vi "Trip Log and Trip Monitor.vi"(8 "error in (no error)":errorcluster, 11 "main ref":T1) -> (0 "error out":errorcluster)   [LabVIEW 2025]
uses:
  controls/LAB-IQ UI Data.ctl
  Traction Loop/Traction Receipe Enum.ctl
  <vilib>/Utility/error.llb/Trim Whitespace One-Sided.vi
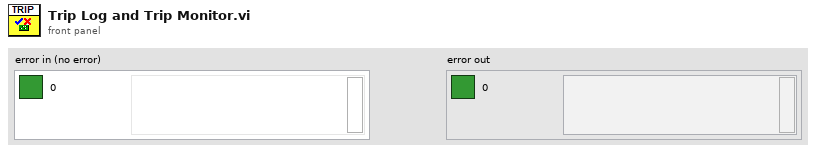
[diagram p1: front panel]
types:
  T1 = typedef "LAB-IQ UI Data.ctl" = cluster{"Main Home Screen":cluster{"GUI":refnum<vi>, "Platform Settings":refnum<vi>, "Configure":refnum<vi>, "Home":refnum<vi>, "EXIT":refnum<vi>, "service 2":refnum<vi>, "MainPage":refnum<vi>, "Analysis":refnum<vi>}, "Platform Settings":cluster{"mm/s  Surge":refnum<vi>, "Update Surge Speed":refnum<vi>, "Drive Error":refnum<vi>, "Disable Axis Jog Soft Limits":refnum<vi>, "mm/s  Sway":refnum<vi>, "Sway and Surge COM Status":refnum<vi>, "Heave COM Status":refnum<vi>, "Enable Platform":refnum<vi>, "Surge Forward Main":refnum<vi>, "Sway Right Main":refnum<vi>, "Sway Left Main":refnum<vi>, "Heave Down Main":refnum<vi>, "Heave Up main":refnum<vi>, "Update Sway Speed":refnum<vi>, "Update Heave Speed":refnum<vi>, "mm/s Heave":refnum<vi>, "mm/sec":refnum<vi>, "mm":refnum<vi>, "Surge Backward Main":refnum<vi>}, "Analysis Screen":cluster{"Analysis Home":refnum<vi>, "Surface Analysis":refnum<vi>, "Imaging":refnum<vi>, "Image Analysis":refnum<vi>, "Post Analysis":refnum<vi>}, "Config Screen":cluster{"Select Load Head":refnum<vi>, "Notes :":refnum<vi>, "FILE":refnum<vi>, "Sample ID :":refnum<vi>, "Operator ID :":refnum<vi>, "Operator Name :":refnum<vi>, "Auto":refnum<vi>}, "Motion Module":cluster{"zNL":refnum<vi>, "NL disp":refnum<vi>, "Rotary Tab":refnum<vi>, "Motion Direction:  3":refnum<vi>, "E.Velocity 2":refnum<vi>, "e.v/ssr 2":refnum<vi>, "Enter Fixed E.Velocity 2":refnum<vi>, "Enter Final SRR 2":refnum<vi>, "Enter initial SRR 2":refnum<vi>, "Enter Fixed SRR 2":refnum<vi>, "Enter the Final E.Velocity (m/s) 2":refnum<vi>, "Enter initial E.Velocity (m/s) 2":refnum<vi>, "Final Speed (RPM) 3":refnum<vi>, "Initial Speed (RPM) 2":refnum<vi>, "Enter the Final Velocity (m/s) 3":refnum<vi>, "Enter initial Velocity (m/s)  3":refnum<vi>, "Ramp Up 2":refnum<vi>, "TEST SELECTION":refnum<vi>, "SPEED SELECTION : ":refnum<vi>, "Angular Oscillation Set":refnum<vi>, "Traction":refnum<vi>, "Step Speed":refnum<vi>, "StepTable For Load-Speed":refnum<vi>, "StepTable For Speed":refnum<vi>, "Surge Forward MM":refnum<vi>, "Surge Backward MM":refnum<vi>, "M3 Image":refnum<vi>, "String 39":refnum<vi>, "Sway Left MM":refnum<vi>, "Sway Right MM":refnum<vi>, "Disable Axis Jog Soft Limits":refnum<vi>, "mm":refnum<vi>, "Heave Down MM":refnum<vi>, "Heave Up MM":refnum<vi>, "Wear Track Diameter (mm)":refnum<vi>, "Set WTD":refnum<vi>, "HomeScratch":refnum<vi>, "HomeRot":refnum<vi>, "PlaceModule":refnum<vi>, "Enter the Angle (Deg)":refnum<vi>, "Enter the Frequency (Hz)":refnum<vi>, "Motion Mode:":refnum<vi>, "LR Sway":refnum<vi>, "Rot Hor":refnum<vi>, "Scratch":refnum<vi>, "LR Cam":refnum<vi>, "MMBack":refnum<vi>, "MMNext":refnum<vi>, "Rot Ver":refnum<vi>, "Rotary Module Selection":refnum<vi>, "calculate rotary":refnum<vi>, "SPEED SELECTION : rotary":refnum<vi>, "Import 2":refnum<vi>, "Save 2":refnum<vi>, "File Path :  2":refnum<vi>, "String 45":refnum<vi>, "StepTable For Speed 3":refnum<vi>, "Enter the Speed(mm/sec)":refnum<vi>, "Enter the Speed(RPM)":refnum<vi>, "Enter Scratch Speed (mm/s):":refnum<vi>, "SwaySpeed Set":refnum<vi>, "Scartch Offset":refnum<vi>, "Motion type:":refnum<vi>, "HomeScratch 2":refnum<vi>, "Enter Scratch length (mm):":refnum<vi>, "Wear Track Diameter":refnum<vi>, "Rotary Speed Exced":refnum<vi>, "Scratch Mode":refnum<vi>, "No of Scratch":refnum<vi>}, "Environmental control":cluster{"Humidity  Status  3":refnum<vi>, "Low Temp  Status  2":refnum<vi>, "TK4 status 2":refnum<vi>, "Stage Temperature":refnum<vi>, "Sample Temperature":refnum<vi>, "Humidity (Amb)":refnum<vi>, "Clear List":refnum<vi>, "Add to list":refnum<vi>, "Wear":refnum<vi>, "Vibration":refnum<vi>, "Humidity (Chamber)":refnum<vi>, "Temperature (Chamber)":refnum<vi>, "ECR ":refnum<vi>, "Temperature (Amb)":refnum<vi>, "Microphone":refnum<vi>, "Acoustic Emission 3":refnum<vi>, "SNext":refnum<vi>, "APBack":refnum<vi>, "Enter the Temperature (°C):":refnum<vi>, "Enter the Stage \nTemperature (°C):":refnum<vi>, "Enter the Humidity (%Rh):":refnum<vi>, "Low Temp":refnum<vi>, "High Temp":refnum<vi>, "Humidity":refnum<vi>, "Sensors Picked":refnum<vi>}, "About Screen":cluster{"Password":refnum<vi>, "Home Service":refnum<vi>, "Advanced Setting":refnum<vi>, "About Tab":refnum<vi>, "ECR Port:":refnum<vi>, "Ramp Port:":refnum<vi>, "Installation/Replacement completed":refnum<vi>, "Loahead":refnum<vi>, "Heave and Surge COM Port:":refnum<vi>, "Sway COM Port:":refnum<vi>, "Temp Modbus:":refnum<vi>, "Humidity Port:":refnum<vi>, "Edit Gain Constants":refnum<vi>, "Save Gain Constants":refnum<vi>}, "Main Screen":cluster{"Main Screen Tab":refnum<vi>, "Angle and Frequency":refnum<vi>, "Stroke (mm)":refnum<vi>, "Angle (Deg)":refnum<vi>, "Main Speed Tab":refnum<vi>, "MTM MOTOR DISPLAY":refnum<vi>, "Disc Speed (m/sec)":refnum<vi>, "Ball Speed (m/sec)":refnum<vi>, "Disc Speed (RPM)":refnum<vi>, "Ball Speed (RPM)":refnum<vi>, "SPEED TAB":refnum<vi>, "Speed (m/sec)":refnum<vi>, "Set Speed (m/sec)":refnum<vi>, "Speed (RPM)":refnum<vi>, "Set Speed":refnum<vi>, "Time Tab":refnum<vi>, "Time ( HH:MM:SS ) 2":refnum<vi>, "Test Duration":refnum<vi>, "Test Duration 4":refnum<vi>, "TEST CYCLE":refnum<vi>, "TOTAL CYCLES":refnum<vi>, "Set Load (N)":refnum<vi>, "Temp Tabs":refnum<vi>, "Heater":refnum<vi>, "TK4 status":refnum<vi>, "ChamberTemp":refnum<vi>, "SetTmp":refnum<vi>, "Controller  Status":refnum<vi>, "ChamberTemp 2":refnum<vi>, "SetTmp 2":refnum<vi>, "Controller  Status 2":refnum<vi>, "ChamberTemp 3":refnum<vi>, "SetTmp 3":refnum<vi>, "Cooling":refnum<vi>, "Load Communication":refnum<vi>, "Ambient \nTemperature":refnum<vi>, "HumCOMStatus":refnum<vi>, "Ambient\n Humidity":refnum<vi>, "Freq (Hz)":refnum<vi>, "Load En":refnum<vi>, "NLt":refnum<vi>, "zNL 2":refnum<vi>, "Humidity On":refnum<vi>, "humidity disp":refnum<vi>, "Set Humidity":refnum<vi>, "NL disp 2":refnum<vi>, "Humidity On 2":refnum<vi>, "humidity disp 2":refnum<vi>, "Set Humidity 2":refnum<vi>, "NL disp 3":refnum<vi>, "AppLoadSeq scratch":refnum<vi>, "Stop Scratch":refnum<vi>, "ClrLog":refnum<vi>, "Trip Log":refnum<vi>, "STOP":refnum<vi>, "Start Test":refnum<vi>, "Test status":refnum<vi>, "AR Led":refnum<vi>, "Data":refnum<vi>, "Health":refnum<vi>, "Sway COM Status":refnum<vi>, "Heave COM Status":refnum<vi>, "Grp Tab":refnum<vi>, "Sub Graph":refnum<vi>, "SD (mm)":refnum<vi>, "Siliding distance Reset Graph":refnum<vi>, "SDGp":refnum<vi>, "Humidity Reset Graph":refnum<vi>, "HumrGp":refnum<vi>, "Acoustic Emission (mV)":refnum<vi>, "Aqucostic Reset Graph":refnum<vi>, "gACQUOS":refnum<vi>, "ECR RESET":refnum<vi>, "ECR":refnum<vi>, "Temperature Reset":refnum<vi>, "Acoustic Emission (mV) 2":refnum<vi>, "Aqucostic Reset Graph 2":refnum<vi>, "gACQUOS 2":refnum<vi>, "ECR RESET 2":refnum<vi>, "ECR 2":refnum<vi>, "Temperature Reset 2":refnum<vi>, "Temperature (deg c)":refnum<vi>, "Speed Reset Graph":refnum<vi>, "Speed Tab":refnum<vi>, "MTM DISC  SPEED":refnum<vi>, "MTM BALL SPEED":refnum<vi>, "speed mm/sec":refnum<vi>, "Hymidity":refnum<vi>, "Humidity Disable trip":refnum<vi>, "CoF Trip  2":refnum<vi>, "Depth Trip":refnum<vi>, "Weart Deapth":refnum<vi>, "Depth Reset Graph":refnum<vi>, "Weart":refnum<vi>, "Depthz":refnum<vi>, "Depth (µm)":refnum<vi>, "WearGp":refnum<vi>, "NL Trip 2":refnum<vi>, "Load pid":refnum<vi>, "Load Disable Trip":refnum<vi>, "Load Reset Graph":refnum<vi>, "NL Display 4":refnum<vi>, "Main Chart 3":refnum<vi>, "BACK":refnum<vi>, "Depth Trip 2":refnum<vi>, "COF TRIP ":refnum<vi>, "Friction Force (N)":refnum<vi>, "FF Reset Graph":refnum<vi>, "FF Disable Trip":refnum<vi>, "FF TRIP":refnum<vi>, "COF Disable Trip":refnum<vi>, "COF Reset Graph":refnum<vi>, "Start Test Temp":refnum<vi>, "zFF":refnum<vi>, "Friction Force (N) Graph":refnum<vi>, "Coefficient of Friction":refnum<vi>, "Scratch Start Test":refnum<vi>, "FF Tab":refnum<vi>, "Cyclic Friction Force (N)":refnum<vi>, "CZ FF":refnum<vi>, "Cyclic Friction Force (N) Graph":refnum<vi>, "Cyclic Coefficient of Friction":refnum<vi>, "Cyclic FF TRIP":refnum<vi>, "Cyclic FF Disable Trip":refnum<vi>, "cyclic COF Disable Trip":refnum<vi>, "cyclic COF TRIP":refnum<vi>, "cyclic COF Reset Graph":refnum<vi>, "Cyclic FF Reset Graph":refnum<vi>, "Test Trip":refnum<vi>, "Multi Scratch Pass":refnum<vi>, "Scratch Start Recording":refnum<vi>}, "Loading":cluster{"Indentation":refnum<vi>, "Reference Sample":refnum<vi>, "Load Cell Communication Slide":refnum<vi>, "com 3":refnum<vi>, "com":refnum<vi>, "DecaForce COM Status":refnum<vi>, "Update":refnum<vi>, "Clear 3":refnum<vi>, "seq":refnum<vi>, "Stribeck table":refnum<vi>, "Stribeck Table  For loading":refnum<vi>, "Loading Mode":refnum<vi>, "Enter the Final Load (N)":refnum<vi>, "Enter the CoF Trip":refnum<vi>, "Enter the Friction Force Trip":refnum<vi>, "Enter the Normal load Trip":refnum<vi>, "Enter the Load  (N)":refnum<vi>, "KiloForce":refnum<vi>, "DecaForce ":refnum<vi>, "MicroForce":refnum<vi>, "LHBack":refnum<vi>, "LHNext":refnum<vi>, "Enter the Loading Rate (N/min)":refnum<vi>, "Message":refnum<vi>, "Warning 2":refnum<vi>, "SSP 0.75":refnum<vi>, "SSP 0.5":refnum<vi>, "SSP 0.3":refnum<vi>, "Warning":refnum<vi>, "gui GIF":refnum<vi>, "Communication is established":refnum<vi>, "AppLoad 4":refnum<vi>, "Multipoint":refnum<vi>, "Load Selection":refnum<vi>}, "PID":cluster{"Ramp MulFac":refnum<vi>, "pulses LoadDiffRamp(2..10)":refnum<vi>, "PulseControlRamp(diff<=3N)":refnum<vi>, "SetLoadDeadband(%) Load(0-10N)":refnum<vi>, "PID gains out delay (microForce)":refnum<vi>, "Ramp":refnum<vi>, "Gain 2":refnum<vi>, "pulses LoadDiff(2..10)":refnum<vi>, "pulses LoadDiff(11..50)":refnum<vi>, "PulseControl(diff<=3N)":refnum<vi>, "SetLoadDeadband(%)  2":refnum<vi>, "Dummy Run":refnum<vi>, "Vertical load (N)":refnum<vi>, "AutoTune":refnum<vi>, "Offset 3 ":refnum<vi>, "apply load":refnum<vi>, "Offset  3":refnum<vi>, "apply load 2":refnum<vi>, "Enter ByPass Load":refnum<vi>, "reinit 3":refnum<vi>, "output range delay":refnum<vi>, "PID gains out delay":refnum<vi>, "Bypass Load":refnum<vi>, "pulsesSent":refnum<vi>, "pulses ":refnum<vi>, "actpid":refnum<vi>, "gFF Rot":refnum<vi>, "pulses LoadDiff(21..1000)":refnum<vi>, "Delay":refnum<vi>, "deadband":refnum<vi>}, "Config Parameters":cluster{"Tab Control 3":refnum<vi>, "Tab Control 19":refnum<vi>, "SAMPLES":refnum<vi>, "Re-initilaize":refnum<vi>, "Filter ON/OFF":refnum<vi>, "TracHomeSurgeOffsetCounts 10MM":refnum<vi>, "TracHomeSwayOffsetCounts 10MM":refnum<vi>, "Acoustic Emission:":refnum<vi>, "Apply Filter (FF)":refnum<vi>, "Filter% 2":refnum<vi>, "Apply Filter (Load)":refnum<vi>, "Filter% ":refnum<vi>, "Sway distance (mm)":refnum<vi>, "Surge distance (mm)":refnum<vi>, "DataSavingLoopDelay(ms)":refnum<vi>, "SAVE 2":refnum<vi>, "Enter Distance":refnum<vi>, "Sway Counts:":refnum<vi>, "Distance (mm): 3":refnum<vi>, "Surge Counts:":refnum<vi>, "Distance (mm): 2":refnum<vi>, "Distance (mm):":refnum<vi>, "Heave Counts:":refnum<vi>, "LRMHomeSurgeOffsetCounts":refnum<vi>, "LRMHomeSwayOffsetCounts":refnum<vi>, "TracHomeSurgeOffsetCounts 20MM":refnum<vi>, "TracHomeSwayOffsetCounts 20MM":refnum<vi>, "RotHomeSwayOffsetCounts":refnum<vi>, "RotHomeSurgeOffsetCounts":refnum<vi>, "Heave distance":refnum<vi>, "Zmm":refnum<vi>, "Heave Pulses/mm":refnum<vi>, "Surge Pulses/mm":refnum<vi>, "Sway Pulses/mm":refnum<vi>, "Heave Pitch":refnum<vi>, "Surge Pitch":refnum<vi>, "Sway Pitch":refnum<vi>, "Heave PPR":refnum<vi>, "Surge PPR":refnum<vi>, "Sway PPR":refnum<vi>, "Tab Control 5":refnum<vi>, "Tab Control 14":refnum<vi>, "Tab Control 26":refnum<vi>, "AE":refnum<vi>, "Heave Loop Delay":refnum<vi>, "Heave PID Speed":refnum<vi>, "Surge Jog Speed":refnum<vi>, "Heave Jog Speed":refnum<vi>, "Sway Loop Delay":refnum<vi>, "Sway PID Speed":refnum<vi>, "Sway Jog Speed":refnum<vi>, "DEPTH TRIP VALUE":refnum<vi>, "LOAD TRIP VALUE":refnum<vi>, "DEPTH TRIP   ENABLE":refnum<vi>, "LOAD TRIP  ENABLE":refnum<vi>, "CYCLIC FF TRIP VALUE":refnum<vi>, "FF TRIP VALUE":refnum<vi>, "CYCLIC CoF TRIP VALUE":refnum<vi>, "COF TRIP VALUE":refnum<vi>, "CYCLIC COF TRIP  ENABLE":refnum<vi>, "CYCLIC FF TRIP  ENABLE":refnum<vi>, "FF TRIP  ENABLE":refnum<vi>, "COF TRIP  ENABLE":refnum<vi>, "JOG TRIP LOAD VALUE (N)":refnum<vi>}, "Loading Com Port":cluster{"ClearAll":refnum<vi>, "Mz(Nm)":refnum<vi>, "My(Nm)":refnum<vi>, "Mx(Nm)":refnum<vi>, "Save Dwell":refnum<vi>, "Mx ":refnum<vi>, "My ":refnum<vi>, "Mz":refnum<vi>, "Fx(N)":refnum<vi>, "Fy(N)":refnum<vi>, "Fz(N)":refnum<vi>, "ZeroAll":refnum<vi>, "Acq Delay (ms)":refnum<vi>, "Burst Delay (ms)":refnum<vi>, "model":refnum<vi>, "SN":refnum<vi>, "FFx(N)":refnum<vi>, "Sensor IP":refnum<vi>, "Port":refnum<vi>, "FFy(N)":refnum<vi>, "Load(N)":refnum<vi>, "delete Handle":refnum<vi>, "Create Handle":refnum<vi>, "ft_data":refnum<vi>, "ft_range":refnum<vi>, "ft_data 2":refnum<vi>, "stop 6":refnum<vi>, "running_flag":refnum<vi>, "ft_udp_handle":refnum<vi>, "get-data-return":refnum<vi>, "get-range-return":refnum<vi>, "zero-return":refnum<vi>, "filter-return":refnum<vi>, "initial-return":refnum<vi>, "deleteHandle-result":refnum<vi>, "Load Cell Temp":refnum<vi>}, "Heave AND Surge":cluster{"SURGE POSE":refnum<vi>, "error out Read":refnum<vi>, "HEAVE POSE":refnum<vi>, "State":refnum<vi>, "Homed":refnum<vi>, "Sequence ID":refnum<vi>, "error out Write":refnum<vi>, "faultCode":refnum<vi>, "Ack ID":refnum<vi>, "SPEED":refnum<vi>, "Distance":refnum<vi>, "Mode Command":refnum<vi>, "Heave and Surge Read":refnum<vi>, "Read Heave Temp":refnum<vi>, "Spare 15":refnum<vi>, "Spare 14":refnum<vi>, "Spare 13":refnum<vi>, "Spare 12":refnum<vi>, "Spare 11":refnum<vi>, "Spare 10":refnum<vi>, "Spare 9":refnum<vi>, "Spare 8":refnum<vi>, "Spare 7":refnum<vi>, "Spare 6":refnum<vi>, "Spare 5":refnum<vi>, "Spare 4":refnum<vi>, "Spare 2":refnum<vi>, "Spare 1":refnum<vi>, "Node Id":refnum<vi>, "Spare 3":refnum<vi>, "SPARE 4":refnum<vi>, "SPARE 3":refnum<vi>, "SPARE 2":refnum<vi>, "SPARE 1":refnum<vi>, "fwMajor":refnum<vi>, "fwMinor":refnum<vi>, "Manual Write":refnum<vi>, "Heave and Surge Write":refnum<vi>, "SPARE 5":refnum<vi>, "Reserved ":refnum<vi>, "SPARE 8":refnum<vi>, "SPARE 6":refnum<vi>, "SPARE 7":refnum<vi>, "SPARE 17":refnum<vi>, "SPARE 16":refnum<vi>, "SPARE 15":refnum<vi>, "SPARE 14":refnum<vi>, "SPARE 13":refnum<vi>, "SPARE 12":refnum<vi>, "SPARE 11":refnum<vi>, "SPARE 10":refnum<vi>, "SPARE 9":refnum<vi>, "System UPTIME":refnum<vi>, "Missed Packets":refnum<vi>, "faultCode Surge Right":refnum<vi>, "faultCode Surge Left":refnum<vi>, "faultCode Heave":refnum<vi>, "UPLINK HEAVE":refnum<vi>, "DOWNLINK HEAVE":refnum<vi>}, "New PID LOGIC":cluster{"Fine Tune Zone":refnum<vi>, "PID SDelay":refnum<vi>, "Max_pos_limit":refnum<vi>, "Min_pos_limit":refnum<vi>, "i_limit":refnum<vi>, "pct_scale":refnum<vi>, "Deadband":refnum<vi>, "Kd":refnum<vi>, "Ki":refnum<vi>, "Kp":refnum<vi>, "Current Position":refnum<vi>, "Set Load":refnum<vi>, "Current Load":refnum<vi>, "Pulse delta":refnum<vi>, "Init Step":refnum<vi>, "Max Step Linit":refnum<vi>, "min_deadband_floor":refnum<vi>, "dynamic_spindle_noise_scalar":refnum<vi>, "min_finetune_floor":refnum<vi>, "filter_alpha":refnum<vi>}, "SWAY ":cluster{"fwMajor":refnum<vi>, "Homed":refnum<vi>, "Rotary POSE":refnum<vi>, "State":refnum<vi>, "SWAY POSE":refnum<vi>, "Ack ID":refnum<vi>, "faultCode":refnum<vi>, "Node Id":refnum<vi>, "fwMinor":refnum<vi>, "Spare 6":refnum<vi>, "Spare 5":refnum<vi>, "Spare 4":refnum<vi>, "Spare 3":refnum<vi>, "Spare 2":refnum<vi>, "Spare 1":refnum<vi>, "Spare 7":refnum<vi>, "SPARE  5":refnum<vi>, "error out Write  SWAY ":refnum<vi>, "error out Read SWAY ":refnum<vi>, "Manual Write SWAY ":refnum<vi>, "SWAY WRITE":refnum<vi>, "SPARE  4":refnum<vi>, "SPARE  3":refnum<vi>, "SPARE 2":refnum<vi>, "SPARE 1":refnum<vi>, "Spare 15":refnum<vi>, "Spare 14":refnum<vi>, "Spare 13":refnum<vi>, "Spare 12":refnum<vi>, "Spare 11":refnum<vi>, "Spare 9":refnum<vi>, "Spare 8":refnum<vi>, "SPEED":refnum<vi>, "Distance":refnum<vi>, "Mode Command":refnum<vi>, "Sequence ID":refnum<vi>, "SWAY READ":refnum<vi>, "Spare 10":refnum<vi>, "Read SWAY Temp":refnum<vi>, "faultCode Sway ":refnum<vi>, "Missed Packets":refnum<vi>, "System UPTIME sway":refnum<vi>, "SPARE 6":refnum<vi>, "SPARE 7":refnum<vi>, "SPARE 9":refnum<vi>, "SPARE 11":refnum<vi>, "SPARE 10":refnum<vi>, "SPARE 8":refnum<vi>, "SPARE 13":refnum<vi>, "SPARE 12":refnum<vi>, "SPARE 17":refnum<vi>, "SPARE 16":refnum<vi>, "SPARE 15":refnum<vi>, "SPARE 14":refnum<vi>, "Reserved":refnum<vi>, "faultCode Rotary":refnum<vi>, "UPLINK SWAY":refnum<vi>, "DOWNLINK SWAY":refnum<vi>}, "Analysis Screen":cluster{"Analysis Home":refnum<vi>, "Refresh 2":refnum<vi>, "MEAN 4":refnum<vi>, "SD 4":refnum<vi>, "VARIANCE 4":refnum<vi>, "MEAN  3":refnum<vi>, "SD  3":refnum<vi>, "VARIANCE  3":refnum<vi>, "MEAN 2":refnum<vi>, "SD  2":refnum<vi>, "VARIANCE 2":refnum<vi>, "MEAN":refnum<vi>, "SD":refnum<vi>, "VARIANCE":refnum<vi>, "File 4 Discription":refnum<vi>, "OPEN 4":refnum<vi>, "File Name 4":refnum<vi>, "OPEN 3":refnum<vi>, "File 3 Discription":refnum<vi>, "File Name 3":refnum<vi>, "Y-AXIS":refnum<vi>, "X-AXIS":refnum<vi>, "XY Graph":refnum<vi>, "File Name 2":refnum<vi>, "File Name 1":refnum<vi>, "OPEN 2":refnum<vi>, "OPEN 1":refnum<vi>, "File 1 Discription ":refnum<vi>, "File 2 Discription":refnum<vi>, "Export":refnum<vi>, "File Format":refnum<vi>}, "Traction":cluster{"faultCode Traction 2":refnum<vi>, "faultCode Traction 1":refnum<vi>, "Missed Packets":refnum<vi>, "System UPTIME Traction":refnum<vi>, "SPARE 17":refnum<vi>, "SPARE 16":refnum<vi>, "SPARE 15":refnum<vi>, "SPARE 14":refnum<vi>, "SPARE 13":refnum<vi>, "SPARE 12":refnum<vi>, "SPARE 11":refnum<vi>, "SPARE 10":refnum<vi>, "SPARE 9":refnum<vi>, "SPARE 8":refnum<vi>, "SPARE 7":refnum<vi>, "SPARE 6":refnum<vi>, "Reserved":refnum<vi>, "SPARE  5":refnum<vi>, "Manual Write TRACTION":refnum<vi>, "TRACTION WRITE":refnum<vi>, "SPARE  4":refnum<vi>, "SPARE  3":refnum<vi>, "SPARE 2":refnum<vi>, "SPARE 1":refnum<vi>, "Spare 7":refnum<vi>, "Spare 6":refnum<vi>, "Spare 5":refnum<vi>, "Spare 4":refnum<vi>, "Spare 2":refnum<vi>, "Spare 1":refnum<vi>, "Node Id":refnum<vi>, "Read TRACTION Temp":refnum<vi>, "fwMinor":refnum<vi>, "fwMajor":refnum<vi>, "faultCode":refnum<vi>, "TRACTION POSE":refnum<vi>, "TRACTION POSE 2":refnum<vi>, "Homed":refnum<vi>, "State":refnum<vi>, "Ack ID":refnum<vi>, "SPEED":refnum<vi>, "Distance":refnum<vi>, "Mode Command":refnum<vi>, "Sequence ID":refnum<vi>, "error out Read TRACTION":refnum<vi>, "error out Write  TRACTION":refnum<vi>, "TRACTION READ":refnum<vi>, "Spare 3":refnum<vi>}, "Traction reciepe":cluster{"SRR Sweep Range (%) Stribeck":refnum<vi>, "Traction Receipe":refnum<vi>, "Total Execution Time":refnum<vi>, "Total Steps":refnum<vi>, "Duration / Step (s)  Stribeck":refnum<vi>, "STRIBECK Fixed SRR List (%)":refnum<vi>, "Duration / Step (s) Traction":refnum<vi>, "SRR Sweep Range (%) traction":refnum<vi>, "Rolling Speed (mm/s)":refnum<vi>, "Temperature Stages (°C)":refnum<vi>, "Ball Load (N)":refnum<vi>, "Lubricant Name":refnum<vi>, "Profile File Name":refnum<vi>, "SET entrainment Velocity":refnum<vi>, "Test Array Size":refnum<vi>, "SRR INDEX [ STRIBECK]":refnum<vi>, "Stribeck Size":refnum<vi>, "SET SRR":refnum<vi>, "ELAPSED TIMER ":refnum<vi>, "BALL SET RPM":refnum<vi>, "DISC SET RPM":refnum<vi>, "SET LOAD":refnum<vi>, "TEMPERATURE READ":refnum<vi>, "SET TEMPERATURE":refnum<vi>, "Traction Size":refnum<vi>, "DISC SPEED (rpm)":refnum<vi>, "BALL SPEED (rpm)":refnum<vi>, "BALL WEAR TRACK":refnum<vi>, "DISC WEARTRACK":refnum<vi>, "SRR INDEX [ TRACTION]":refnum<vi>, "Start Index Type":refnum<vi>, "Enum - Menu":refnum<vi>, "Ball (mm/sec)":refnum<vi>, "Disc (mm/sec)":refnum<vi>}, "Traction Control":cluster{"HomeTraction":refnum<vi>, "Demo Mode Display":refnum<vi>, "Traction Message":refnum<vi>, "Traction Step Update Details":refnum<vi>, "Main Tab sequence for selection":refnum<vi>, "Ramp Tab":refnum<vi>, "e.v/ssr":refnum<vi>, "Enter Fixed E.Velocity":refnum<vi>, "Enter Final SRR":refnum<vi>, "Enter initial SRR":refnum<vi>, "Enter Fixed SRR":refnum<vi>, "Enter the Final E.Velocity (m/s)":refnum<vi>, "Enter initial E.Velocity (m/s)":refnum<vi>, "Ball WTD":refnum<vi>, "E.Velocity":refnum<vi>, "Enter the Final Velocity (m/s)":refnum<vi>, "Enter initial Velocity (m/s)":refnum<vi>, "Ramp Up   Disc":refnum<vi>, "Initial DiscSpeed (RPM)":refnum<vi>, "Final Speed (RPM) Ball":refnum<vi>, "Final Speed (RPM)":refnum<vi>, "Initial Speed (RPM) Ball":refnum<vi>, "Enter the Final Velocity (m/s) Ball":refnum<vi>, "Enter initial Velocity (m/s) Ball":refnum<vi>, "Ramp Up":refnum<vi>, "ExceedBallSpeed step":refnum<vi>, "ExceedDiscSpeed":refnum<vi>, "BallSpeed Exceed Indication":refnum<vi>, "Apply":refnum<vi>, "SPEED SELECTION : MTM":refnum<vi>, "SPEED SELECTION : MTM 2":refnum<vi>, "TEST SELECTION (MTM)":refnum<vi>, "MTM Test Selection":refnum<vi>, "File Path Tab":refnum<vi>, "File Path String":refnum<vi>, "Save":refnum<vi>, "Save  2":refnum<vi>, "Import ":refnum<vi>, "File Path :":refnum<vi>, "Step Sequence Indication Tab":refnum<vi>, "Step Sequence Indication":refnum<vi>, "Calculate Step":refnum<vi>, "StepTable":refnum<vi>, "ExceedDiscSpeed  Cinstant Speed":refnum<vi>, "ExceedBallSpeed Constant":refnum<vi>, "TEST SELECTION (MTM) 2":refnum<vi>, "SPEED SELECTION : MTM 3":refnum<vi>, "MTM Test Selection 2":refnum<vi>, "Enter the Speed (m/sec): ":refnum<vi>, "Enter the Speed (m/sec):  2":refnum<vi>, "Enter the Speed (RPM):":refnum<vi>, "Lower Spped ":refnum<vi>, "Upper":refnum<vi>, "Enter the Speed (RPM):Ball":refnum<vi>, "Disc Motion Direction: ":refnum<vi>, "Ball Motion Direction :":refnum<vi>, "Motion Mode: ":refnum<vi>, "Wear Track Diameter (mm) ":refnum<vi>, "Disc Speed Indicator":refnum<vi>, "ExceedBallSpeed":refnum<vi>}, "Acquostic":cluster{"Last Config Rejected ":refnum<vi>, "rx command count":refnum<vi>, "Current Filter Id":refnum<vi>, "Isolated Gain":refnum<vi>, "DAQ Status":refnum<vi>, "error out":refnum<vi>, "error in (no error)":refnum<vi>, "Uplink Packet":refnum<vi>, "data out":refnum<vi>, "Downlink Packet":refnum<vi>, "Signal Energy":refnum<vi>, "Amplitude db_AE":refnum<vi>, "Peak Amplitude":refnum<vi>, "AE Ring-Down Counts":refnum<vi>, "Gains":refnum<vi>, "Manual Write Acquostic":refnum<vi>}}
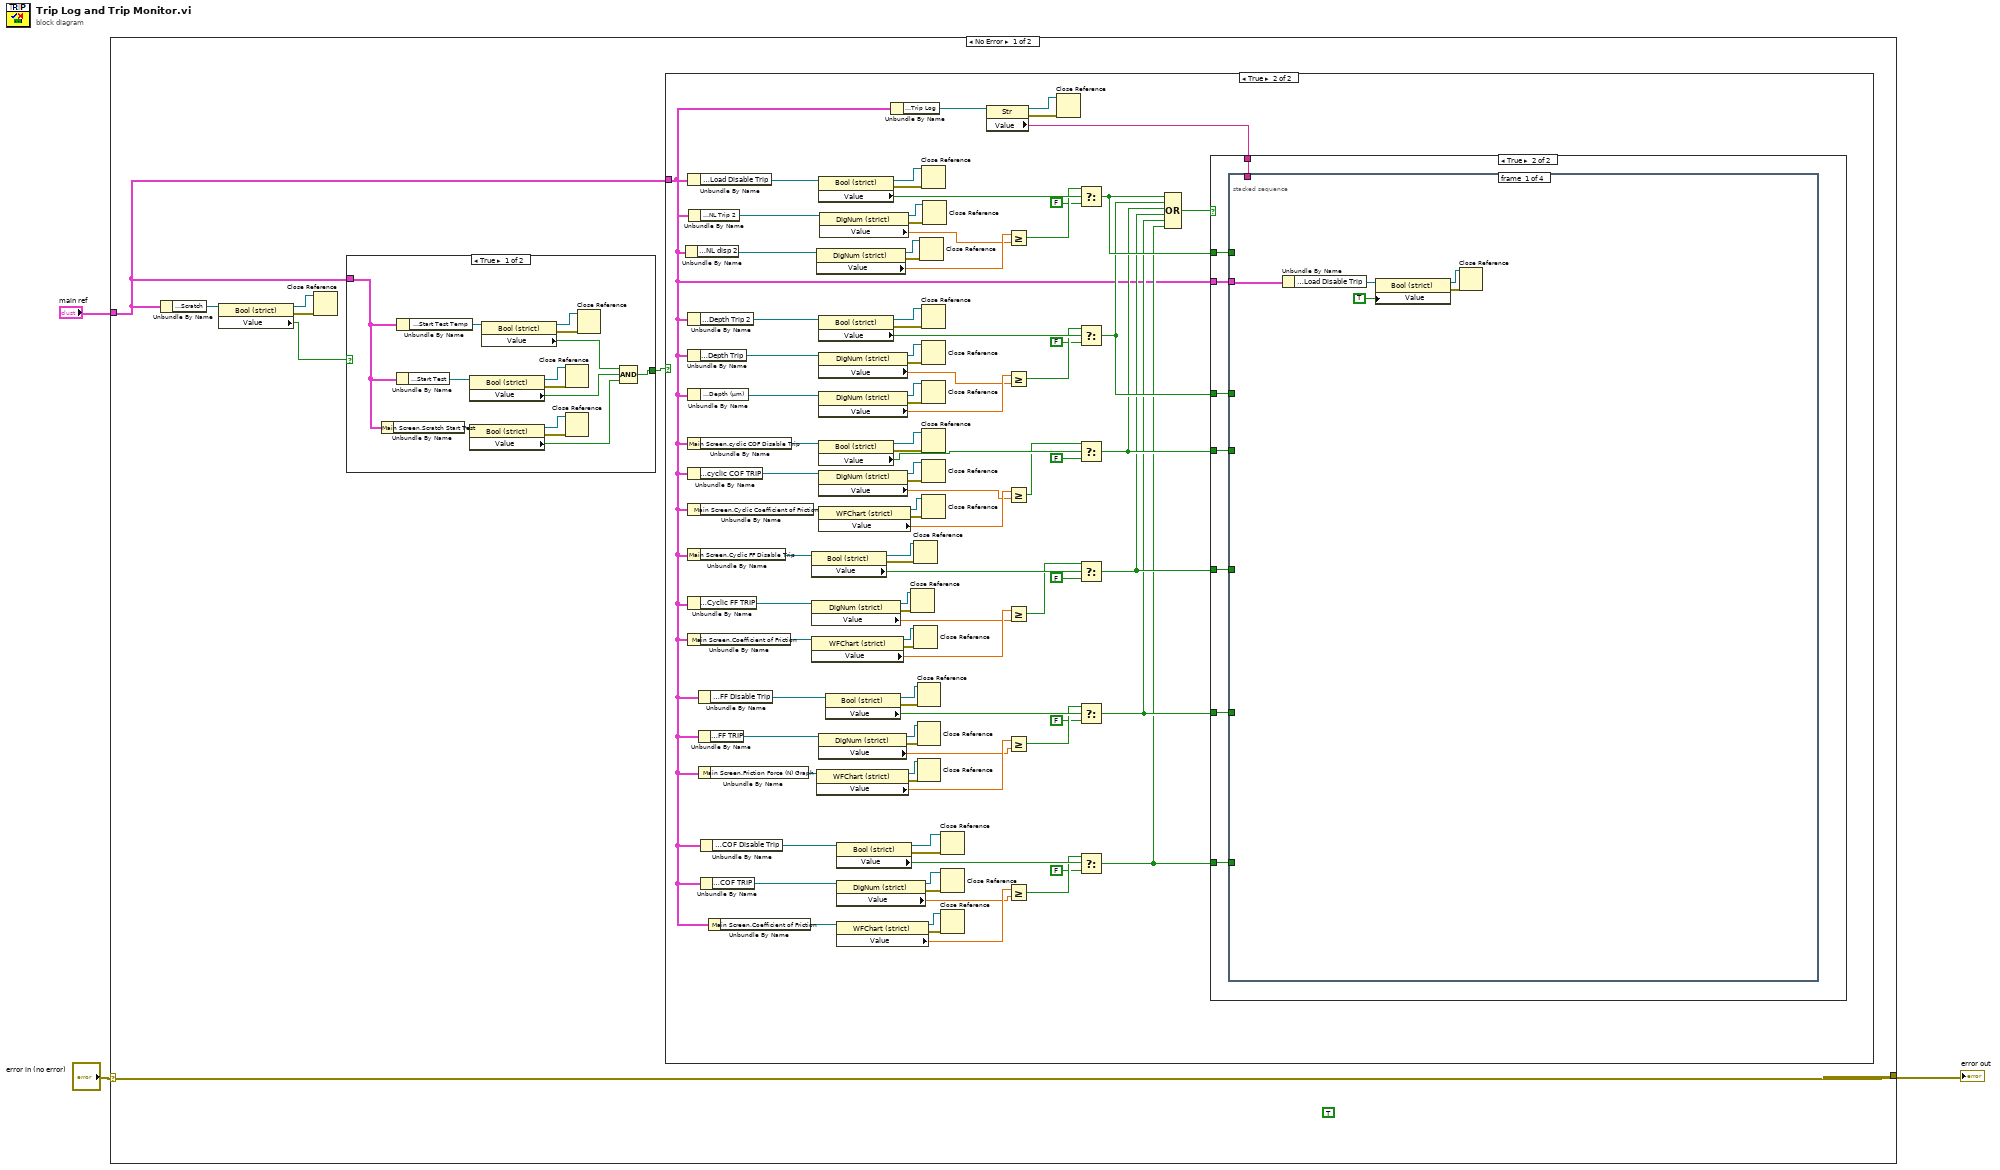
[diagram p0: block diagram]
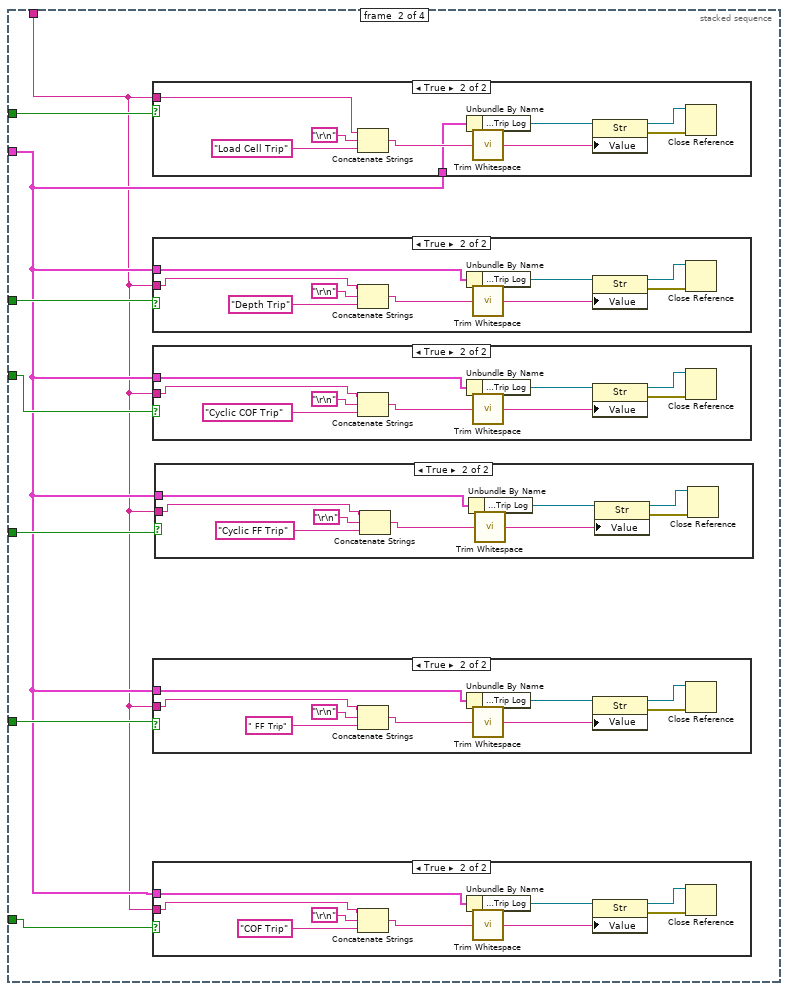
[diagram p4: hidden frame]
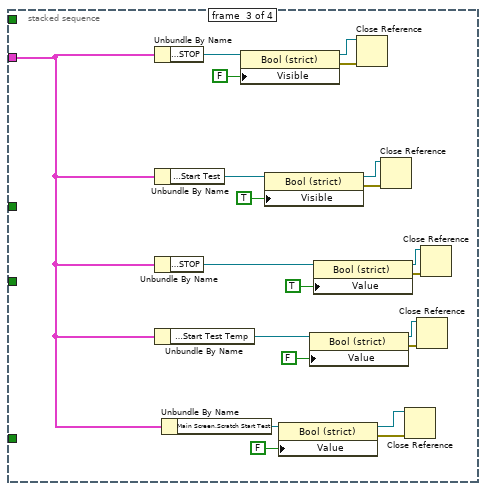
[diagram p11: hidden frame]
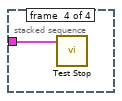
[diagram p12: hidden frame]
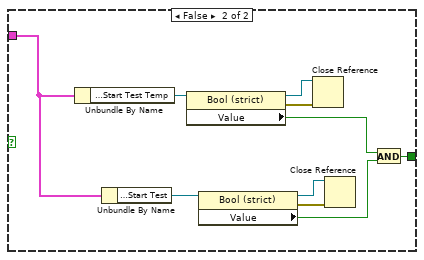
[diagram p13: hidden frame]
diagram:
  n1 = case shown="No Error" "error in (no error)" {
    selector: "error in (no error)" -> [w10 _]
    tunnel: [w10 _] -> w2
    tunnel: "main ref" -> [w9 _]
    frame No Error {
      (unwired) TRUE
      n2 = Unbundle By Name(w9) -> ("Motion Module.Scratch"=w7:refnum<vi>)
      n3 = property class="Bool (strict)"(reference=w7) -> (reference out=w8:refnum<vi>, error out=w6:errorcluster, "Value"=w5:bool)  [unwired: 1 in]
      n4 = Close Reference(reference=w8, error in (no error)=w6) -> ()  [unwired: 1 out]
      n5 = case shown="True" w5 {
        tunnel: w9 -> [w205 w221]
        tunnel: [w209 w219] -> w4
        frame True {
          n6 = Unbundle By Name(w205) -> ("Main Screen.Scratch Start Test"=w207:refnum<vi>)
          n7 = Unbundle By Name(w205) -> ("Main Screen.Start Test"=w213:refnum<vi>)
          n8 = Unbundle By Name(w205) -> ("Main Screen.Start Test Temp"=w216:refnum<vi>)
          n9 = property class="Bool (strict)"(reference=w213) -> (reference out=w212:refnum<vi>, error out=w214:errorcluster, "Value"=w210:bool)  [unwired: 1 in]
          n10 = property class="Bool (strict)"(reference=w207) -> (reference out=w208:refnum<vi>, error out=w206:errorcluster, "Value"=w204:bool)  [unwired: 1 in]
          n11 = property class="Bool (strict)"(reference=w216) -> (reference out=w217:refnum<vi>, error out=w215:errorcluster, "Value"=w211:bool)  [unwired: 1 in]
          n12 = Close Reference(reference=w212, error in (no error)=w214) -> ()  [unwired: 1 out]
          n13 = Close Reference(reference=w208, error in (no error)=w206) -> ()  [unwired: 1 out]
          n14 = Close Reference(reference=w217, error in (no error)=w215) -> ()  [unwired: 1 out]
          n15 = Compound Arithmetic op=AND(w211, w210, w204) -> (w209:bool)
        }
        frame False {
          n16 = Unbundle By Name(w221) -> ("Main Screen.Start Test Temp"=w226:refnum<vi>)
          n17 = Unbundle By Name(w221) -> ("Main Screen.Start Test"=w223:refnum<vi>)
          n18 = property class="Bool (strict)"(reference=w226) -> (reference out=w227:refnum<vi>, error out=w225:errorcluster, "Value"=w220:bool)  [unwired: 1 in]
          n19 = property class="Bool (strict)"(reference=w223) -> (reference out=w222:refnum<vi>, error out=w224:errorcluster, "Value"=w218:bool)  [unwired: 1 in]
          n20 = Close Reference(reference=w227, error in (no error)=w225) -> ()  [unwired: 1 out]
          n21 = Close Reference(reference=w222, error in (no error)=w224) -> ()  [unwired: 1 out]
          n22 = And(x=w220, y=w218) -> (x .and. y?=w219:bool)
        }
      }
      n23 = case shown="True" w4 {
        tunnel: w9 -> [_ w12]
        frame False {
        }
        frame True {
          n24 = Unbundle By Name(w12) -> ("Main Screen.NL disp 2"=w106:refnum<vi>)
          n25 = Unbundle By Name(w12) -> ("Main Screen.Load Disable Trip"=w83:refnum<vi>)
          n26 = Unbundle By Name(w12) -> ("Main Screen.Depth Trip 2"=w78:refnum<vi>)
          n27 = Unbundle By Name(w12) -> ("Main Screen.Depth Trip"=w81:refnum<vi>)
          n28 = Unbundle By Name(w12) -> ("Main Screen.Depth (µm)"=w103:refnum<vi>)
          n29 = Unbundle By Name(w12) -> ("Main Screen.cyclic COF Disable Trip"=w75:refnum<vi>)
          n30 = Unbundle By Name(w12) -> ("Main Screen.cyclic COF TRIP"=w72:refnum<vi>)
          n31 = Unbundle By Name(w12) -> ("Main Screen.Cyclic Coefficient of Friction"=w100:refnum<vi>)
          n32 = Unbundle By Name(w12) -> ("Main Screen.Cyclic FF Disable Trip"=w66:refnum<vi>)
          n33 = Unbundle By Name(w12) -> ("Main Screen.Cyclic FF TRIP"=w69:refnum<vi>)
          n34 = Unbundle By Name(w12) -> ("Main Screen.Coefficient of Friction"=w97:refnum<vi>)
          n35 = Unbundle By Name(w12) -> ("Main Screen.NL Trip 2"=w86:refnum<vi>)
          n36 = Unbundle By Name(w12) -> ("Main Screen.FF Disable Trip"=w93:refnum<vi>)
          n37 = Unbundle By Name(w12) -> ("Main Screen.FF TRIP"=w64:refnum<vi>)
          n38 = Unbundle By Name(w12) -> ("Main Screen.Friction Force (N) Graph"=w59:refnum<vi>)
          n39 = Unbundle By Name(w12) -> ("Main Screen.COF TRIP"=w55:refnum<vi>)
          n40 = Unbundle By Name(w12) -> ("Main Screen.COF Disable Trip"=w56:refnum<vi>)
          n41 = Unbundle By Name(w12) -> ("Main Screen.Coefficient of Friction"=w92:refnum<vi>)
          n42 = property class="Bool (strict)"(reference=w66) -> (reference out=w67:refnum<vi>, error out=w65:errorcluster, "Value"=w49:bool)  [unwired: 1 in]
          n43 = property class="DigNum (strict)"(reference=w69) -> (reference out=w68:refnum<vi>, error out=w70:errorcluster, "Value"=w36:dbl)  [unwired: 1 in]
          n44 = property class="WFChart (strict)"(reference=w97) -> (reference out=w98:refnum<vi>, error out=w96:errorcluster, "Value"=w37:dbl)  [unwired: 1 in]
          n45 = property class="DigNum (strict)"(reference=w106) -> (reference out=w89:refnum<vi>, error out=w105:errorcluster, "Value"=w46:dbl)  [unwired: 1 in]
          n46 = property class="WFChart (strict)"(reference=w59) -> (reference out=w60:refnum<vi>, error out=w61:errorcluster, "Value"=w34:dbl)  [unwired: 1 in]
          n47 = property class="DigNum (strict)"(reference=w64) -> (reference out=w63:refnum<vi>, error out=w62:errorcluster, "Value"=w33:dbl)  [unwired: 1 in]
          n48 = property class="Bool (strict)"(reference=w83) -> (reference out=w85:refnum<vi>, error out=w84:errorcluster, "Value"=w52:bool)  [unwired: 1 in]
          n49 = property class="Bool (strict)"(reference=w78) -> (reference out=w79:refnum<vi>, error out=w77:errorcluster, "Value"=w51:bool)  [unwired: 1 in]
          n50 = property class="DigNum (strict)"(reference=w81) -> (reference out=w80:refnum<vi>, error out=w82:errorcluster, "Value"=w42:dbl)  [unwired: 1 in]
          n51 = property class="DigNum (strict)"(reference=w103) -> (reference out=w104:refnum<vi>, error out=w102:errorcluster, "Value"=w43:dbl)  [unwired: 1 in]
          n52 = property class="Bool (strict)"(reference=w75) -> (reference out=w76:refnum<vi>, error out=w74:errorcluster, "Value"=w50:bool)  [unwired: 1 in]
          n53 = property class="DigNum (strict)"(reference=w72) -> (reference out=w71:refnum<vi>, error out=w73:errorcluster, "Value"=w39:dbl)  [unwired: 1 in]
          n54 = property class="WFChart (strict)"(reference=w100) -> (reference out=w99:refnum<vi>, error out=w101:errorcluster, "Value"=w40:dbl)  [unwired: 1 in]
          n55 = property class="DigNum (strict)"(reference=w86) -> (reference out=w88:refnum<vi>, error out=w87:errorcluster, "Value"=w45:dbl)  [unwired: 1 in]
          n56 = property class="Bool (strict)"(reference=w93) -> (reference out=w94:refnum<vi>, error out=w95:errorcluster, "Value"=w48:bool)  [unwired: 1 in]
          n57 = property class="Bool (strict)"(reference=w56) -> (reference out=w58:refnum<vi>, error out=w57:errorcluster, "Value"=w47:bool)  [unwired: 1 in]
          n58 = property class="DigNum (strict)"(reference=w55) -> (reference out=w53:refnum<vi>, error out=w54:errorcluster, "Value"=w30:dbl)  [unwired: 1 in]
          n59 = property class="WFChart (strict)"(reference=w92) -> (reference out=w90:refnum<vi>, error out=w91:errorcluster, "Value"=w31:dbl)  [unwired: 1 in]
          n60 = Unbundle By Name(w12) -> ("Main Screen.Trip Log"=w13:refnum<vi>)
          n61 = Close Reference(reference=w68, error in (no error)=w70) -> ()  [unwired: 1 out]
          n62 = Close Reference(reference=w67, error in (no error)=w65) -> ()  [unwired: 1 out]
          n63 = Close Reference(reference=w98, error in (no error)=w96) -> ()  [unwired: 1 out]
          n64 = Close Reference(reference=w94, error in (no error)=w95) -> ()  [unwired: 1 out]
          n65 = Close Reference(reference=w63, error in (no error)=w62) -> ()  [unwired: 1 out]
          n66 = Close Reference(reference=w60, error in (no error)=w61) -> ()  [unwired: 1 out]
          n67 = Close Reference(reference=w89, error in (no error)=w105) -> ()  [unwired: 1 out]
          n68 = Close Reference(reference=w85, error in (no error)=w84) -> ()  [unwired: 1 out]
          n69 = Close Reference(reference=w79, error in (no error)=w77) -> ()  [unwired: 1 out]
          n70 = Close Reference(reference=w80, error in (no error)=w82) -> ()  [unwired: 1 out]
          n71 = Close Reference(reference=w104, error in (no error)=w102) -> ()  [unwired: 1 out]
          n72 = Close Reference(reference=w76, error in (no error)=w74) -> ()  [unwired: 1 out]
          n73 = Close Reference(reference=w71, error in (no error)=w73) -> ()  [unwired: 1 out]
          n74 = Close Reference(reference=w99, error in (no error)=w101) -> ()  [unwired: 1 out]
          n75 = Close Reference(reference=w88, error in (no error)=w87) -> ()  [unwired: 1 out]
          n76 = Close Reference(reference=w58, error in (no error)=w57) -> ()  [unwired: 1 out]
          n77 = Close Reference(reference=w53, error in (no error)=w54) -> ()  [unwired: 1 out]
          n78 = Close Reference(reference=w90, error in (no error)=w91) -> ()  [unwired: 1 out]
          n79 = property class="Str"(reference=w13) -> (reference out=w14:refnum<vi>, error out=w15:errorcluster, "Value"=w11:string)  [unwired: 1 in]
          n80 = Greater Or Equal?(x=w46, y=w45) -> (x >= y?=w44:bool)
          n81 = Greater Or Equal?(x=w43, y=w42) -> (x >= y?=w41:bool)
          n82 = Greater Or Equal?(x=w40, y=w39) -> (x >= y?=w38:bool)
          n83 = Greater Or Equal?(x=w37, y=w36) -> (x >= y?=w35:bool)
          n84 = Greater Or Equal?(x=w34, y=w33) -> (x >= y?=w32:bool)
          n85 = Greater Or Equal?(x=w31, y=w30) -> (x >= y?=w29:bool)
          n86 = Close Reference(reference=w14, error in (no error)=w15) -> ()  [unwired: 1 out]
          n87 = Select(t=w44, s=w52, f=FALSE) -> (s? t:f=w21:bool)
          n88 = Select(t=w41, s=w51, f=FALSE) -> (s? t:f=w20:bool)
          n89 = Select(t=w38, s=w50, f=FALSE) -> (s? t:f=w19:bool)
          n90 = Select(t=w35, s=w49, f=FALSE) -> (s? t:f=w18:bool)
          n91 = Select(t=w32, s=w48, f=FALSE) -> (s? t:f=w17:bool)
          n92 = Select(t=w29, s=w47, f=FALSE) -> (s? t:f=w16:bool)
          n93 = Compound Arithmetic op=OR(w21, w20, w19, w18, w17, w16) -> (w22:bool)
          n94 = case shown="True" w22 {
            tunnel: w12 -> [_ w114]
            tunnel: w21 -> [_ w113]
            tunnel: w20 -> [_ w112]
            tunnel: w19 -> [_ w111]
            tunnel: w18 -> [_ w110]
            tunnel: w17 -> [_ w109]
            tunnel: w16 -> [_ w108]
            tunnel: w11 -> [_ w107]
            frame False {
            }
            frame True {
              n95 = stacked-sequence {
                tunnel: w114 -> [w116 w121 w182 w203]
                tunnel: w113 -> [_ w127 _ _]
                tunnel: w112 -> [_ w126 _ _]
                tunnel: w111 -> [_ w125 _ _]
                tunnel: w110 -> [_ w124 _ _]
                tunnel: w109 -> [_ w123 _ _]
                tunnel: w108 -> [_ w122 _ _]
                tunnel: w107 -> [_ w120 _ _]
                frame #0 {
                  n96 = Unbundle By Name(w116) -> ("Main Screen.Load Disable Trip"=w117:refnum<vi>)
                  n97 = property class="Bool (strict)"(reference=w117, "Value"=TRUE) -> (reference out=w119:refnum<vi>, error out=w118:errorcluster)  [unwired: 1 in]
                  n98 = Close Reference(reference=w119, error in (no error)=w118) -> ()  [unwired: 1 out]
                }
                frame #1 {
                  n99 = case shown="True" w127 {
                    tunnel: w121 -> [_ w175]
                    tunnel: w120 -> [_ w173]
                    frame False {
                    }
                    frame True {
                      n100 = Concatenate Strings(w173, "\r\n", "Load Cell Trip" ("string")) -> (w177:string)
                      n101 = Unbundle By Name(w175) -> ("Main Screen.Trip Log"=w174:refnum<vi>)
                      n102 = call <vilib>:"Trim Whitespace.vi"("string"=w177) -> ("trimmed string"=w176:string)  [unwired: 1 in]
                      n103 = property class="Str"(reference=w174, "Value"=w176) -> (reference out=w178:refnum<vi>, error out=w179:errorcluster)  [unwired: 1 in]
                      n104 = Close Reference(reference=w178, error in (no error)=w179) -> ()  [unwired: 1 out]
                    }
                  }
                  n105 = case shown="True" w126 {
                    tunnel: w121 -> [_ w165]
                    tunnel: w120 -> [_ w164]
                    frame False {
                    }
                    frame True {
                      n106 = Concatenate Strings(w164, "\r\n", "Depth Trip" ("string")) -> (w168:string)
                      n107 = Unbundle By Name(w165) -> ("Main Screen.Trip Log"=w166:refnum<vi>)
                      n108 = call <vilib>:"Trim Whitespace.vi"("string"=w168) -> ("trimmed string"=w167:string)  [unwired: 1 in]
                      n109 = property class="Str"(reference=w166, "Value"=w167) -> (reference out=w169:refnum<vi>, error out=w170:errorcluster)  [unwired: 1 in]
                      n110 = Close Reference(reference=w169, error in (no error)=w170) -> ()  [unwired: 1 out]
                    }
                  }
                  n111 = case shown="True" w125 {
                    tunnel: w121 -> [_ w156]
                    tunnel: w120 -> [_ w155]
                    frame False {
                    }
                    frame True {
                      n112 = Concatenate Strings(w155, "\r\n", "Cyclic COF Trip" ("string")) -> (w159:string)
                      n113 = Unbundle By Name(w156) -> ("Main Screen.Trip Log"=w157:refnum<vi>)
                      n114 = call <vilib>:"Trim Whitespace.vi"("string"=w159) -> ("trimmed string"=w158:string)  [unwired: 1 in]
                      n115 = property class="Str"(reference=w157, "Value"=w158) -> (reference out=w160:refnum<vi>, error out=w161:errorcluster)  [unwired: 1 in]
                      n116 = Close Reference(reference=w160, error in (no error)=w161) -> ()  [unwired: 1 out]
                    }
                  }
                  n117 = case shown="True" w123 {
                    tunnel: w121 -> [_ w138]
                    tunnel: w120 -> [_ w137]
                    frame False {
                    }
                    frame True {
                      n118 = Concatenate Strings(w137, "\r\n", " FF Trip" ("string")) -> (w141:string)
                      n119 = Unbundle By Name(w138) -> ("Main Screen.Trip Log"=w139:refnum<vi>)
                      n120 = call <vilib>:"Trim Whitespace.vi"("string"=w141) -> ("trimmed string"=w140:string)  [unwired: 1 in]
                      n121 = property class="Str"(reference=w139, "Value"=w140) -> (reference out=w142:refnum<vi>, error out=w143:errorcluster)  [unwired: 1 in]
                      n122 = Close Reference(reference=w142, error in (no error)=w143) -> ()  [unwired: 1 out]
                    }
                  }
                  n123 = case shown="True" w122 {
                    tunnel: w121 -> [_ w129]
                    tunnel: w120 -> [_ w128]
                    frame False {
                    }
                    frame True {
                      n124 = Concatenate Strings(w128, "\r\n", "COF Trip" ("string")) -> (w132:string)
                      n125 = Unbundle By Name(w129) -> ("Main Screen.Trip Log"=w130:refnum<vi>)
                      n126 = call <vilib>:"Trim Whitespace.vi"("string"=w132) -> ("trimmed string"=w131:string)  [unwired: 1 in]
                      n127 = property class="Str"(reference=w130, "Value"=w131) -> (reference out=w133:refnum<vi>, error out=w134:errorcluster)  [unwired: 1 in]
                      n128 = Close Reference(reference=w133, error in (no error)=w134) -> ()  [unwired: 1 out]
                    }
                  }
                  n129 = case shown="True" w124 {
                    tunnel: w121 -> [_ w147]
                    tunnel: w120 -> [_ w146]
                    frame False {
                    }
                    frame True {
                      n130 = Concatenate Strings(w146, "\r\n", "Cyclic FF Trip" ("string")) -> (w150:string)
                      n131 = Unbundle By Name(w147) -> ("Main Screen.Trip Log"=w148:refnum<vi>)
                      n132 = call <vilib>:"Trim Whitespace.vi"("string"=w150) -> ("trimmed string"=w149:string)  [unwired: 1 in]
                      n133 = property class="Str"(reference=w148, "Value"=w149) -> (reference out=w151:refnum<vi>, error out=w152:errorcluster)  [unwired: 1 in]
                      n134 = Close Reference(reference=w151, error in (no error)=w152) -> ()  [unwired: 1 out]
                    }
                  }
                }
                frame #2 {
                  n135 = Unbundle By Name(w182) -> ("Main Screen.STOP"=w197:refnum<vi>)
                  n136 = Unbundle By Name(w182) -> ("Main Screen.Start Test"=w200:refnum<vi>)
                  n137 = Unbundle By Name(w182) -> ("Main Screen.STOP"=w191:refnum<vi>)
                  n138 = Unbundle By Name(w182) -> ("Main Screen.Start Test Temp"=w190:refnum<vi>)
                  n139 = Unbundle By Name(w182) -> ("Main Screen.Scratch Start Test"=w185:refnum<vi>)
                  n140 = property class="Bool (strict)"(reference=w197, "Visible"=FALSE) -> (reference out=w187:refnum<vi>, error out=w196:errorcluster)  [unwired: 1 in]
                  n141 = property class="Bool (strict)"(reference=w200, "Visible"=TRUE) -> (reference out=w202:refnum<vi>, error out=w201:errorcluster)  [unwired: 1 in]
                  n142 = property class="Bool (strict)"(reference=w185, "Value"=FALSE) -> (reference out=w186:refnum<vi>, error out=w184:errorcluster)  [unwired: 1 in]
                  n143 = property class="Bool (strict)"(reference=w190, "Value"=FALSE) -> (reference out=w188:refnum<vi>, error out=w189:errorcluster)  [unwired: 1 in]
                  n144 = property class="Bool (strict)"(reference=w191, "Value"=TRUE) -> (reference out=w193:refnum<vi>, error out=w192:errorcluster)  [unwired: 1 in]
                  n145 = Close Reference(reference=w187, error in (no error)=w196) -> ()  [unwired: 1 out]
                  n146 = Close Reference(reference=w202, error in (no error)=w201) -> ()  [unwired: 1 out]
                  n147 = Close Reference(reference=w186, error in (no error)=w184) -> ()  [unwired: 1 out]
                  n148 = Close Reference(reference=w188, error in (no error)=w189) -> ()  [unwired: 1 out]
                  n149 = Close Reference(reference=w193, error in (no error)=w192) -> ()  [unwired: 1 out]
                }
                frame #3 {
                  n150 = call "Test Stop.vi"("Data Cluster"=w203) -> ()  [unwired: 10 in, 1 out]
                }
              }
            }
          }
        }
      }
    }
    frame Error {
    }
  }
  "error out" <- w2
